vi "CircPoly.vi"(10 "NumSides":dbl, 11 "Diameter":dbl) -> (3 "VertexArray":T1[](array[typedef]))   [LabVIEW 2014]
uses:
  TypeDefs/Point2DwSlope.ctl
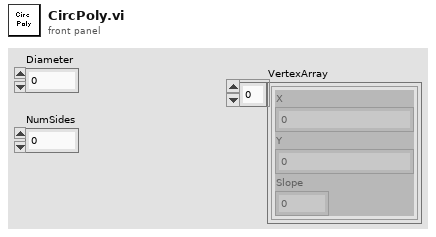
[diagram p1: front panel]
types:
  T1 = typedef "Point2DwSlope.ctl" = cluster{"X":sgl, "Y":sgl, "Slope":dbl}
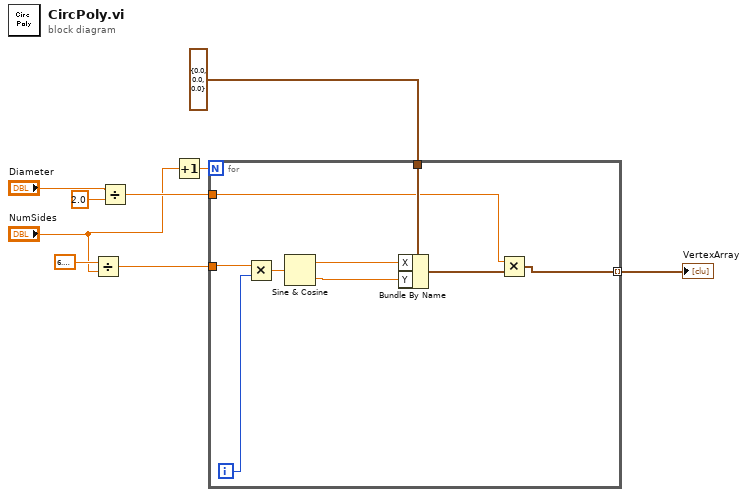
[diagram p0: block diagram]
diagram:
  n1 = Divide(x=6.283185307179586, y="NumSides") -> (x/y=w3:dbl)
  n2 = Divide(x="Diameter", y=2.0) -> (x/y=w5:dbl)
  n3 = Increment(x="NumSides") -> (x+1=w2:dbl)
  n4 = for {
    N: w2 -> [_]
    tunnel: w3 -> [w18]
    tunnel: T1 {"X"=0.0, "Y"=0.0, "Slope"=0.0} ("Point2D") -> [w15]
    tunnel: [w10] -> w8 mode=indexing
    tunnel: w5 -> [w11]
    i -> [w17]
    n5 = Multiply(x=w18, y=w17) -> (x*y=w16:dbl)
    n6 = Sine & Cosine(0:w16) -> (1:w14:dbl, 2:w13:dbl)
    n7 = Bundle By Name(cluster=w15, "X"=w14, "Y"=w13) -> (w12:T1)
    n8 = Multiply(x=w11, y=w12) -> (x*y=w10:cluster{"X":dbl, "Y":dbl, "Slope":dbl})
  }
  "VertexArray" <- w8
